vi "CHROMA Build Command.vi"(7 "Build Type":T1, 8 "Error In":errorcluster, 9 "String":string, 10 "Value":dbl, 11 "Partial Command":string) -> (0 "Error Out":errorcluster, 3 "Chroma Command":string)   [LabVIEW 2020]
uses:
  Type Definition/CHROMA Build CMD Type.ctl
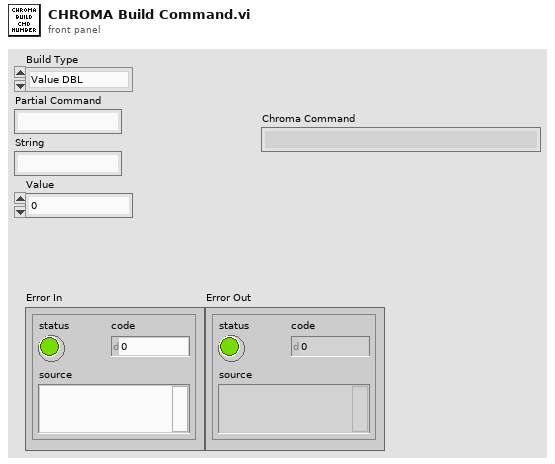
[diagram p1: front panel]
types:
  T1 = typedef "CHROMA Build CMD Type.ctl" = enum16{"Value DBL", "Value I32", "String"}
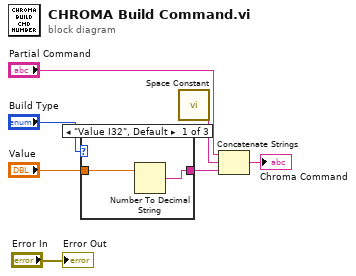
[diagram p0: block diagram]
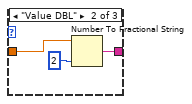
[diagram p2: hidden frame]
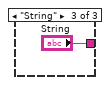
[diagram p3: hidden frame]
diagram:
  n1 = case shown="\"Value I32\", Default" "Build Type" {
    tunnel: [w9 w12 "String"] -> w6
    tunnel: "Value" -> [w8 w11 _]
    frame "Value I32", Default {
      n2 = Number To Decimal String(number=w8) -> (decimal integer string=w9:string)  [unwired: 1 in]
    }
    frame "Value DBL" {
      n3 = Number To Fractional String(number=w11, precision (6)=i16 2) -> (F-format string=w12:string)  [unwired: 2 in]
    }
    frame "String" {
    }
  }
  n4 = call <vilib>:"Space Constant.vi"() -> ("String"=w5:string)
  n5 = Concatenate Strings("Partial Command", w5, w6) -> (→"Chroma Command":string)
  "Error Out" <- "Error In"
